vi "FrontPanel.vi"() -> ()   [LabVIEW 2014]
panel:
  in  "stop":bool
  in  "Click ok after selection":bool
  in  "select from the list":T1(ring)
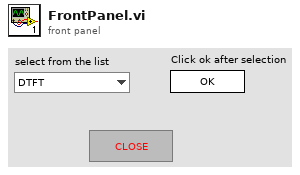
[diagram p1: front panel]
types:
  T1 = enum16{"DTFT", "Periodicity", "Linearity", "Time Shifting", "Convolution", "Time Scaling", "Time Reversal"}
  T2 = enum32{"Invalid", "Standard", "Closed", "Hidden", "Minimized", "Maximized"}
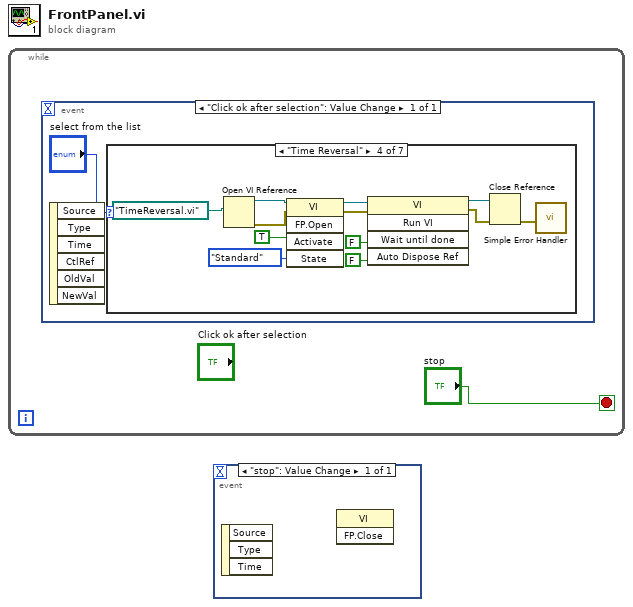
[diagram p0: block diagram]
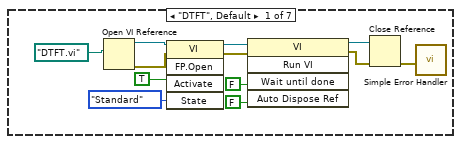
[diagram p2: hidden frame]
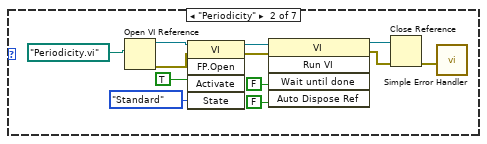
[diagram p3: hidden frame]
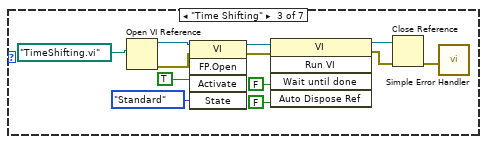
[diagram p4: hidden frame]
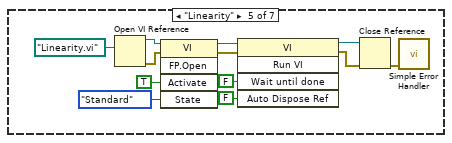
[diagram p5: hidden frame]
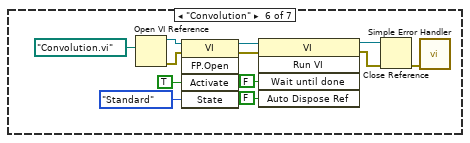
[diagram p6: hidden frame]
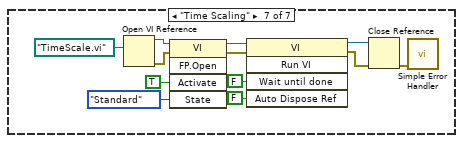
[diagram p7: hidden frame]
diagram:
  n1 = while {
    stop <- "stop" stop-if-true
    n2 = event shown="[0] \"Click ok after selection\": Value Change" {
      selector: _ -> [_]
      dyn-events: _ -> [_]
      timeout: _ -> [_]
      event "Click ok after selection": Value Change {
        n3 = event-data() -> ()  [unwired: 1 in, 6 out]
        n4 = case shown="\"Time Reversal\"" "select from the list" {
          frame "DTFT", Default {
            n5 = Open VI Reference(vi path=path "DTFT.vi") -> (vi reference=w13:refnum<vi>, error out=w12:errorcluster)  [unwired: 5 in]
            n6 = invoke class="VI" method="FP.Open"(reference=w13, error in=w12, "Activate"=TRUE ("Activate?"), "State"=T2."Standard") -> (reference out=w9:refnum<vi>, error out=w8:errorcluster)  [unwired: 1 in, 3 out]
            n7 = invoke class="VI" method="Run VI"(reference=w9, error in=w8, "Wait until done"=FALSE ("Wait Until Done"), "Auto Dispose Ref"=FALSE ("Auto Dispose Reference")) -> (reference out=w5:refnum<vi>, error out=w4:errorcluster)  [unwired: 1 in, 3 out]
            n8 = Close Reference(reference=w5, error in (no error)=w4) -> (error out=w3:errorcluster)
            n9 = call <vilib>:"Simple Error Handler.vi"("error in (no error)"=w3) -> ()  [unwired: 4 in, 5 out]
          }
          frame "Periodicity" {
            n10 = Open VI Reference(vi path=path "Periodicity.vi") -> (vi reference=w25:refnum<vi>, error out=w24:errorcluster)  [unwired: 5 in]
            n11 = invoke class="VI" method="FP.Open"(reference=w25, error in=w24, "Activate"=TRUE ("Activate?"), "State"=T2."Standard") -> (reference out=w21:refnum<vi>, error out=w20:errorcluster)  [unwired: 1 in, 3 out]
            n12 = invoke class="VI" method="Run VI"(reference=w21, error in=w20, "Wait until done"=FALSE ("Wait Until Done"), "Auto Dispose Ref"=FALSE ("Auto Dispose Reference")) -> (reference out=w17:refnum<vi>, error out=w16:errorcluster)  [unwired: 1 in, 3 out]
            n13 = Close Reference(reference=w17, error in (no error)=w16) -> (error out=w15:errorcluster)
            n14 = call <vilib>:"Simple Error Handler.vi"("error in (no error)"=w15) -> ()  [unwired: 4 in, 5 out]
          }
          frame "Time Shifting" {
            n15 = Open VI Reference(vi path=path "TimeShifting.vi") -> (vi reference=w37:refnum<vi>, error out=w36:errorcluster)  [unwired: 5 in]
            n16 = invoke class="VI" method="FP.Open"(reference=w37, error in=w36, "Activate"=TRUE ("Activate?"), "State"=T2."Standard") -> (reference out=w33:refnum<vi>, error out=w32:errorcluster)  [unwired: 1 in, 3 out]
            n17 = invoke class="VI" method="Run VI"(reference=w33, error in=w32, "Wait until done"=FALSE ("Wait Until Done"), "Auto Dispose Ref"=FALSE ("Auto Dispose Reference")) -> (reference out=w29:refnum<vi>, error out=w28:errorcluster)  [unwired: 1 in, 3 out]
            n18 = Close Reference(reference=w29, error in (no error)=w28) -> (error out=w27:errorcluster)
            n19 = call <vilib>:"Simple Error Handler.vi"("error in (no error)"=w27) -> ()  [unwired: 4 in, 5 out]
          }
          frame "Time Reversal" {
            n20 = Open VI Reference(vi path=path "TimeReversal.vi") -> (vi reference=w49:refnum<vi>, error out=w48:errorcluster)  [unwired: 5 in]
            n21 = invoke class="VI" method="FP.Open"(reference=w49, error in=w48, "Activate"=TRUE ("Activate?"), "State"=T2."Standard") -> (reference out=w45:refnum<vi>, error out=w44:errorcluster)  [unwired: 1 in, 3 out]
            n22 = invoke class="VI" method="Run VI"(reference=w45, error in=w44, "Wait until done"=FALSE ("Wait Until Done"), "Auto Dispose Ref"=FALSE ("Auto Dispose Reference")) -> (reference out=w41:refnum<vi>, error out=w40:errorcluster)  [unwired: 1 in, 3 out]
            n23 = Close Reference(reference=w41, error in (no error)=w40) -> (error out=w39:errorcluster)
            n24 = call <vilib>:"Simple Error Handler.vi"("error in (no error)"=w39) -> ()  [unwired: 4 in, 5 out]
          }
          frame "Linearity" {
            n25 = Open VI Reference(vi path=path "Linearity.vi") -> (vi reference=w61:refnum<vi>, error out=w60:errorcluster)  [unwired: 5 in]
            n26 = invoke class="VI" method="FP.Open"(reference=w61, error in=w60, "Activate"=TRUE ("Activate?"), "State"=T2."Standard") -> (reference out=w57:refnum<vi>, error out=w56:errorcluster)  [unwired: 1 in, 3 out]
            n27 = invoke class="VI" method="Run VI"(reference=w57, error in=w56, "Wait until done"=FALSE ("Wait Until Done"), "Auto Dispose Ref"=FALSE ("Auto Dispose Reference")) -> (reference out=w53:refnum<vi>, error out=w52:errorcluster)  [unwired: 1 in, 3 out]
            n28 = Close Reference(reference=w53, error in (no error)=w52) -> (error out=w51:errorcluster)
            n29 = call <vilib>:"Simple Error Handler.vi"("error in (no error)"=w51) -> ()  [unwired: 4 in, 5 out]
          }
          frame "Convolution" {
            n30 = Open VI Reference(vi path=path "Convolution.vi") -> (vi reference=w73:refnum<vi>, error out=w72:errorcluster)  [unwired: 5 in]
            n31 = invoke class="VI" method="FP.Open"(reference=w73, error in=w72, "Activate"=TRUE ("Activate?"), "State"=T2."Standard") -> (reference out=w69:refnum<vi>, error out=w68:errorcluster)  [unwired: 1 in, 3 out]
            n32 = invoke class="VI" method="Run VI"(reference=w69, error in=w68, "Wait until done"=FALSE ("Wait Until Done"), "Auto Dispose Ref"=FALSE ("Auto Dispose Reference")) -> (reference out=w65:refnum<vi>, error out=w64:errorcluster)  [unwired: 1 in, 3 out]
            n33 = Close Reference(reference=w65, error in (no error)=w64) -> (error out=w63:errorcluster)
            n34 = call <vilib>:"Simple Error Handler.vi"("error in (no error)"=w63) -> ()  [unwired: 4 in, 5 out]
          }
          frame "Time Scaling" {
            n35 = Open VI Reference(vi path=path "TimeScale.vi") -> (vi reference=w85:refnum<vi>, error out=w84:errorcluster)  [unwired: 5 in]
            n36 = invoke class="VI" method="FP.Open"(reference=w85, error in=w84, "Activate"=TRUE ("Activate?"), "State"=T2."Standard") -> (reference out=w81:refnum<vi>, error out=w80:errorcluster)  [unwired: 1 in, 3 out]
            n37 = invoke class="VI" method="Run VI"(reference=w81, error in=w80, "Wait until done"=FALSE ("Wait Until Done"), "Auto Dispose Ref"=FALSE ("Auto Dispose Reference")) -> (reference out=w77:refnum<vi>, error out=w76:errorcluster)  [unwired: 1 in, 3 out]
            n38 = Close Reference(reference=w77, error in (no error)=w76) -> (error out=w75:errorcluster)
            n39 = call <vilib>:"Simple Error Handler.vi"("error in (no error)"=w75) -> ()  [unwired: 4 in, 5 out]
          }
        }
      }
    }
  }
  n40 = event shown="[0] \"stop\": Value Change" {
    selector: _ -> [_]
    dyn-events: _ -> [_]
    timeout: _ -> [_]
    event "stop": Value Change {
      n41 = event-data() -> ()  [unwired: 1 in, 3 out]
      n42 = invoke class="VI" method="FP.Close"() -> ()  [unwired: 3 in, 3 out]
    }
  }
